vi "ELTA_channel_mapping.vi"(10 "Ch_2_cal.":i32=16, 11 "Ch_1_ref":i32=16) -> (3 "Operating \nChannel(s)":bool[][](array[boolean]))   [LabVIEW 2023, in "ELTA.lvlib"]
uses:
  ELTA.lvlib
panel:
  # "0"
  # "16"
  # "15"
  # "23"
  # "7"
  # "8"
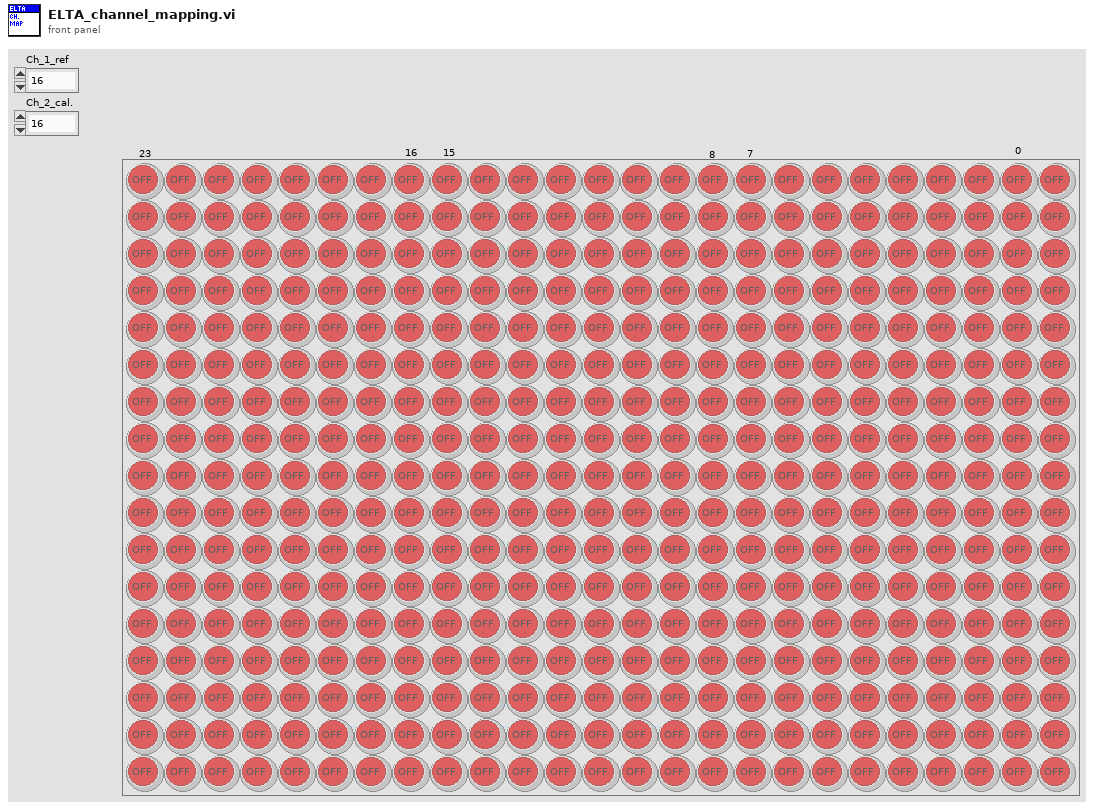
[diagram p1: front panel]
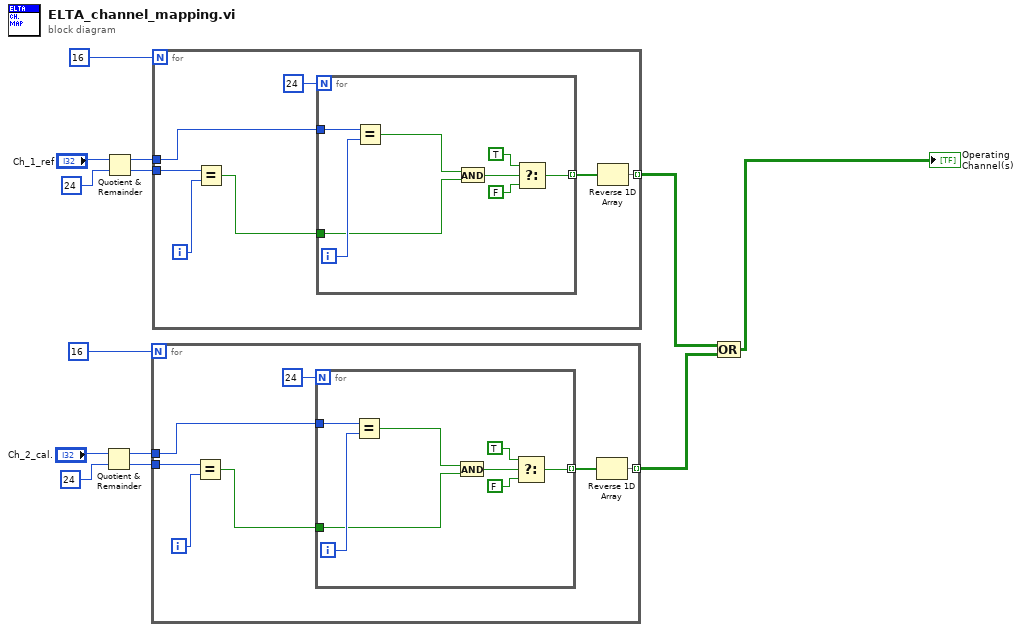
[diagram p0: block diagram]
diagram:
  n1 = Quotient & Remainder(x="Ch_2_cal.", y=24) -> (x-y*floor(x/y)=w4:i32, floor(x/y)=w5:i32)
  n2 = Quotient & Remainder(x="Ch_1_ref", y=24) -> (x-y*floor(x/y)=w13:i32, floor(x/y)=w12:i32)
  n3 = for {
    N: 16 -> [_]
    tunnel: [w14] -> w2 mode=indexing
    tunnel: w4 -> [w16]
    tunnel: w5 -> [w18]
    i -> [w17]
    n4 = Equal?(x=w18, y=w17) -> (x = y?=w15:bool)
    n5 = for {
      N: 24 -> [_]
      tunnel: [w23] -> w19 mode=indexing
      tunnel: w15 -> [w26]
      tunnel: w16 -> [w28]
      i -> [w27]
      n6 = Equal?(x=w28, y=w27) -> (x = y?=w21:bool)
      n7 = And(x=w21, y=w26) -> (x .and. y?=w22:bool)
      n8 = Select(t=TRUE, s=w22, f=FALSE) -> (s? t:f=w23:bool)
    }
    n9 = Reverse 1D Array(array=w19) -> (reversed array=w14:bool[])
  }
  n10 = for {
    N: 16 -> [_]
    tunnel: [w29] -> w3 mode=indexing
    tunnel: w13 -> [w31]
    tunnel: w12 -> [w33]
    i -> [w32]
    n11 = Equal?(x=w33, y=w32) -> (x = y?=w30:bool)
    n12 = for {
      N: 24 -> [_]
      tunnel: [w38] -> w34 mode=indexing
      tunnel: w30 -> [w41]
      tunnel: w31 -> [w43]
      i -> [w42]
      n13 = Equal?(x=w43, y=w42) -> (x = y?=w36:bool)
      n14 = And(x=w36, y=w41) -> (x .and. y?=w37:bool)
      n15 = Select(t=TRUE, s=w37, f=FALSE) -> (s? t:f=w38:bool)
    }
    n16 = Reverse 1D Array(array=w34) -> (reversed array=w29:bool[])
  }
  n17 = Compound Arithmetic op=OR(w3, w2) -> (→"Operating \nChannel(s)":bool[][])
